vi "PVCAM_Uninit.vi"(8 "error in (no error)":errorcluster) -> (0 "error out":errorcluster, 3 "return value":i16)   [LabVIEW 2021]
uses:
  pvcam64.dll
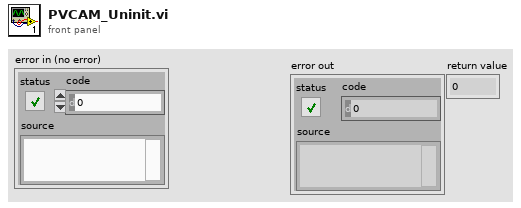
[diagram p1: front panel]
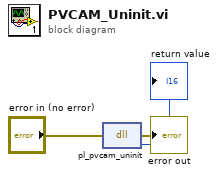
[diagram p0: block diagram]
diagram:
  n1 = dll-call lib="pvcam64.dll" fn="pl_pvcam_uninit"(error in="error in (no error)") -> (error out=→"error out":errorcluster, "return type"=→"return value":i16)  [unwired: 2 in, 1 out]
